vi "Execute.vi"(8 "error in (no error)":errorcluster, 11 "Node in":refnum<class "Test Boolean.lvclass">) -> (0 "error out":errorcluster, 1 "Status":T1, 3 "Node out":refnum<class "Test Boolean.lvclass">)   [LabVIEW 2021, in "BT AbsType.lvlib" / "Test Boolean.lvclass"]
uses:
  Test Boolean.lvclass
  C:/Users/Tim/Documents/GitHub/LV_Behaviour_Tree/BT Abstract Type/abs_Type Leaf/abs_Type Leaf.lvclass
  Source/Support/Nodes/abs_Node/Status.ctl
  <vilib>/TSA/Abstract Data Classes/Abs_Types/Boolean/Abs_Boolean.lvclass
  C:/Program Files (x86)/National Instruments/LabVIEW 2021/vi.lib/TSA/Abstract Data Classes/Abs_Types/Type/Abs_Type.lvclass
  abs_Type Leaf/abs_Type Leaf.lvclass/abs_Type Leaf.ctl
  abs_Type Leaf/Properties/Read Value Class.vi
  abs_Type Leaf/Properties/Write Value Class.vi
  abs_Type Leaf/abs_Type Leaf.lvclass
  <vilib>/TSA/Abstract Data Classes/Abs_Types/Type/Abs_Type.lvclass
  Source/Support/Nodes/abs_Node/bt_Node.lvclass
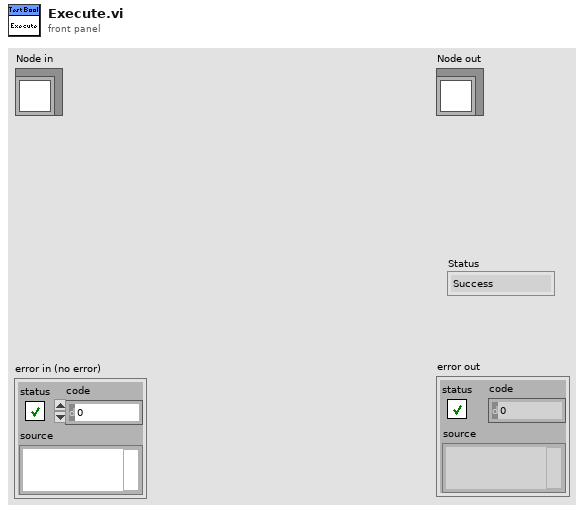
[diagram p1: front panel]
types:
  T1 = typedef "BT.lvlib/bt_Node.lvclass/Status.ctl" = enum16{"Success", "Failure", "Running"}
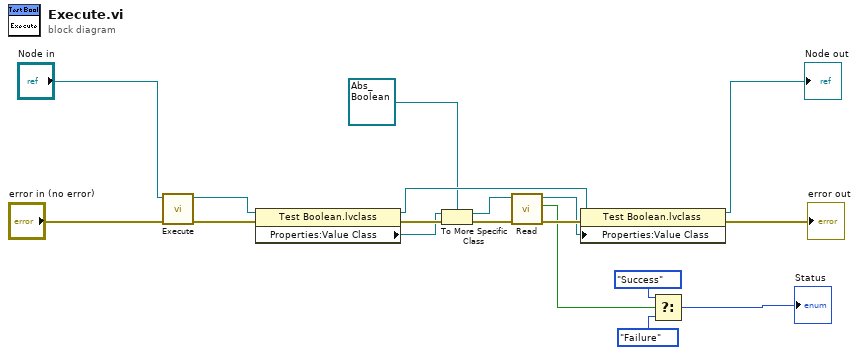
[diagram p0: block diagram]
diagram:
  n1 = call-parent "Execute.vi"("error in (no error)"="error in (no error)", "Node in"="Node in") -> ("error out"=w13:errorcluster, "Node out"=w12:refnum<class "Test Boolean.lvclass">)  [unwired: 7 in, 1 out]
  n2 = property class="Test Boolean.lvclass"(reference=w12, error in=w13) -> (reference out=w11:refnum<class "Test Boolean.lvclass">, error out=w7:errorcluster, "Properties:Value Class"=w5:refnum<class "Abs_Type.lvclass">)
  n3 = To More Specific Class(target class=refnum<class "Abs_Boolean.lvclass"> refnum ("Boolean in"), reference=w5, error in=w7) -> (specific class reference=w3:refnum<class "Abs_Boolean.lvclass">, error out=w6:errorcluster)
  n4 = call-dynamic "Read.vi"("error in (no error)"=w6, "Boolean in"=w3) -> ("error out"=w10:errorcluster, "Boolean"=w8:bool, "Boolean out"=w9:refnum<class "Abs_Boolean.lvclass">)  [unwired: 7 in]
  n5 = property class="Test Boolean.lvclass"(reference=w11, error in=w10, "Properties:Value Class"=w9) -> (reference out=→"Node out":refnum<class "Test Boolean.lvclass">, error out=→"error out":errorcluster)
  n6 = Select(t=Status."Success" ("Status"), s=w8, f=Status."Failure" ("Status")) -> (s? t:f=→"Status":T1)
